vi "Labo-3-VI.vi-a-réutiliser.vi"() -> ()   [LabVIEW 2020]
uses:
  <instrlib>/Agilent 34401/Public/Data/Read (Single Point).vi
  <instrlib>/Agilent E363X Series/Agilent E363X Series.lvlib
  <instrlib>/Agilent 34401/Agilent 34401.lvlib
panel:
  out "XY Graph":cluster{"Y":dbl[], "Y":dbl[]}[](graph) caption="Graphe XY"
  in  "Plage tension":dbl(slide) scale=0.0..4.0
  out "Courant":dbl
  in  "Incrément tension":dbl
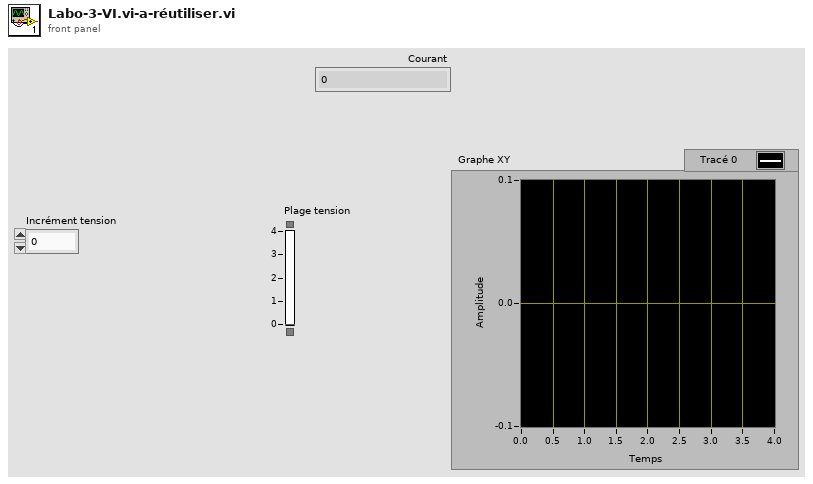
[diagram p1: front panel]
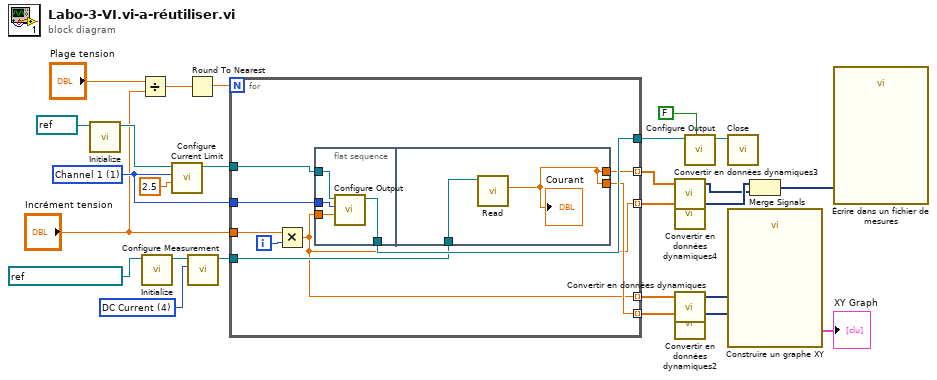
[diagram p0: block diagram]
diagram:
  w21 = u16 4 items=["DC Voltage", "AC Voltage", "2 - Wire Resistance", "4 - Wire Resistance", "DC Current", "AC Current", "Frequency", "Period", "Continuity", "Diode Checking", "VDC:VDC Ratio", "Temperature", "Capacitance"] ("Function (0: DC Voltage)")
  w18 = 1 items=["Channel 1"=1, "Channel 2"=2, "Channel 3"=3] ("Channel (1: Channel 1)")
  n1 = call <instrlib>:"Initialize.vi"("VISA resource name"=refnum<visa-resource-name> "GPIB0::5::INSTR") -> ("VISA resource name out"=w25:refnum<visa-resource-name>)  [unwired: 9 in, 1 out]
  n2 = Divide(x="Plage tension", y="Incrément tension") -> (x/y=w12:dbl)
  n3 = call <instrlib>:"Initialize.vi"("VISA resource name"=refnum<visa-resource-name> "GPIB0::22::INSTR") -> ("VISA resource name out"=w22:refnum<visa-resource-name>)  [unwired: 9 in, 1 out]
  n4 = call <instrlib>:"Configure Current Limit.vi"("Current Limit (0.0 A)"=2.5, "Channel (1: Channel 1)"=w18, "VISA resource name"=w25) -> ("VISA resource name out"=w17:refnum<visa-resource-name>)  [unwired: 7 in, 1 out]
  n5 = Round To Nearest(number=w12) -> (nearest integer value=w11:dbl)
  n6 = call <instrlib>:"Configure Measurement.vi"("Function (0: DC Voltage)"=w21, "VISA resource name"=w22) -> ("VISA resource name out"=w15:refnum<visa-resource-name>)  [unwired: 8 in, 1 out]
  n7 = for {
    N: w11 -> [_]
    tunnel: w18 -> [w35]
    tunnel: w17 -> [w34]
    tunnel: [w33] -> w16
    tunnel: w15 -> [w32]
    tunnel: "Incrément tension" -> [w31]
    tunnel: [w27] -> w9 mode=indexing
    tunnel: [w29] -> w7 mode=indexing
    tunnel: [w28] -> w5 mode=indexing
    tunnel: [w27] -> w4 mode=indexing
    i -> [w30]
    n8 = Multiply(x=w31, y=w30) -> (x*y=w27:dbl)
    n9 = flat-sequence {
      tunnel: w35 -> [w39]
      tunnel: w34 -> [w38]
      tunnel: [w37] -> w33
      tunnel: w27 -> [w36]
      tunnel: w32 -> [w41]
      tunnel: [w40] -> w29
      tunnel: [w40] -> w28
      frame #0 {
        n10 = call <instrlib>:"Configure Output.vi"("Voltage Level (0.0 V)"=w36, "Channel (1: Channel 1)"=w39, "VISA resource name"=w38) -> ("VISA resource name out"=w37:refnum<visa-resource-name>)  [unwired: 7 in, 1 out]
      }
      frame #1 {
        n11 = call-poly <instrlib>:"Read.vi"("VISA resource name"=w41) -> ("Measurement"=w40:dbl)  [unwired: 8 in, 2 out]
        "Courant" <- w40
      }
    }
  }
  n12 = call "Convertir en données dynamiques3"("Array"=w5) -> ("Dynamic Data Type"=w1:dynamicdata)  [unwired: 3 in]
  n13 = call "Convertir en données dynamiques4"("Array"=w4) -> ("Dynamic Data Type"=w2:dynamicdata)  [unwired: 3 in]
  n14 = call "Convertir en données dynamiques"("Array"=w9) -> ("Dynamic Data Type"=w8:dynamicdata)  [unwired: 3 in]
  n15 = call "Convertir en données dynamiques2"("Array"=w7) -> ("Dynamic Data Type"=w6:dynamicdata)  [unwired: 3 in]
  n16 = call <instrlib>:"Configure Output.vi"("Enable Output (T: Enable)"=FALSE, "VISA resource name"=w16) -> ("VISA resource name out"=w19:refnum<visa-resource-name>)  [unwired: 8 in, 1 out]
  n17 = call <instrlib>:"Close.vi"("VISA resource name"=w19) -> ()  [unwired: 10 in, 1 out]
  n18 = call "Construire un graphe XY"("Y Input"=w6, "X Input"=w8) -> ("XY Graph"=→"XY Graph":cluster{"X":dbl[], "Y":dbl[]}[])  [unwired: 8 in, 1 out]
  n19 = Merge Signals(w2, w1) -> (w3:dynamicdata)
  n20 = call "Écrire dans un fichier de mesures"("Signals"=w3) -> ()  [unwired: 16 in, 3 out]
